vi "CalculateNumberDenisty.vi"(10 "Sample Molar Mass (g/mol)":dbl, 11 "Sample Density (g/cm^3)":dbl) -> (3 "Number Density (ions/cm^3)":dbl)   [LabVIEW 2012]
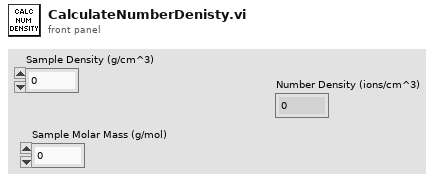
[diagram p1: front panel]
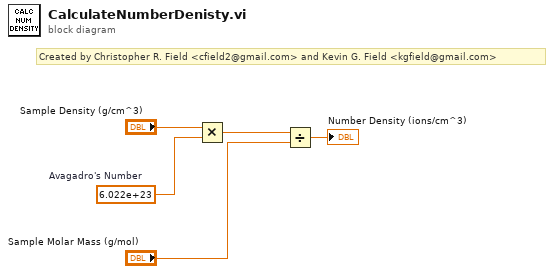
[diagram p0: block diagram]
diagram:
  w4 = 6.022e+23  # Avagadro's Number
  # "Created by Christopher R. Field <cfield2@gmail.com> and Kevin G. Field <kgfield@gmail.com>"
  n1 = Multiply(x="Sample Density (g/cm^3)", y=w4) -> (x*y=w3:dbl)
  n2 = Divide(x=w3, y="Sample Molar Mass (g/mol)") -> (x/y=→"Number Density (ions/cm^3)":dbl)
